vi "Begin.vi"(8 "error in":errorcluster) -> (0 "error out":errorcluster)   [LabVIEW 2016]
doc: "Called before other user functions, this VI is expected to open initial I/O refnums, load in file data, and do all program initialization. Notice that the <B>error out</B> terminal is simply used for data flow. Wiring it to other structures or subVIs ensures that this VI runs first."
uses:
  <vilib>/Rock Robotics/WPI/DriverStation/WPI_DriverStationRobotMode2.ctl
  <vilib>/Rock Robotics/WPI/SafetyOutput/WPI_SafetyOutputConfigMenu.ctl
  <vilib>/Rock Robotics/WPI/Joystick/WPI_JoystickDeviceEnum.ctl
  <vilib>/Rock Robotics/WPI/ThirdParty/CanMotor/TalonSRX/WPI_CANTalonSRX_APIControlMode.ctl
  <vilib>/Rock Robotics/WPI/Solenoid/WPI_SolenoidChannel.ctl
  <vilib>/Rock Robotics/SystemInterfaces/spilib/spi_bus.ctl
  <vilib>/Rock Robotics/WPI/ThirdParty/CanMotor/TalonSRX/WPI_CANTalonSRX_APIFeedbackSelect.ctl
  <vilib>/Rock Robotics/SystemInterfaces/DIO/FPGA_DIOChannel.ctl
  Robot Global Data.vi
  <vilib>/Rock Robotics/WPI/RobotDrive/WPI_RobotDriveOpen4MotorWithExistingMotors.vi
  <vilib>/Rock Robotics/WPI/Solenoid/WPI_SolenoidOpenDouble.vi
  <vilib>/Rock Robotics/WPI/Solenoid/WPI_SolenoidOpenSingle.vi
  <vilib>/Rock Robotics/WPI/Gyro/WPI_GyroXRS450_SPI_Open.vi
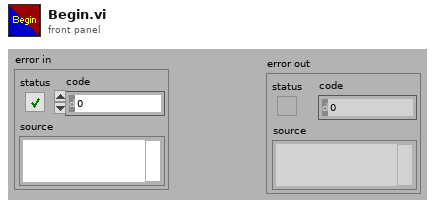
[diagram p1: front panel]
types:
  T1 = typedef "FPGA_DIOChannel.ctl" = enum8{"DIO 0", "DIO 1", "DIO 2", "DIO 3", "DIO 4", "DIO 5", "DIO 6", "DIO 7", "DIO 8", "DIO 9", "DIO MXP 0", "DIO MXP 1", "DIO MXP 2", "DIO MXP 3", "DIO MXP 4", "DIO MXP 5", "DIO MXP 6", "DIO MXP 7", "DIO MXP 8", "DIO MXP 9", "DIO MXP 10", "DIO MXP 11", "DIO MXP 12", "DIO MXP 13", "DIO MXP 14", "DIO MXP 15", "SPI Port CS1", "SPI Port CS2", "SPI Port CS3", "SPI Port MISO", "SPI Port MOSI", "Invalid"}
  T2 = typedef "WPI_CANTalonSRX_APIFeedbackSelect.ctl" = enum16{"Digital Quadrature Encoder", "Analog Potentiometer", "Analog Encoder", "Count on Quad-A (Rising-Edge)", "Count on Quad-A (Falling-Edge)", "CTR Magnetic Enc (Absolute)", "CTR Magnetic Enc (Relative)", "Pulse Width"}
  T3 = typedef "spi_bus.ctl" = enum16{"SPI On-Board, CS0", "SPI On-Board, CS1", "SPI On-Board, CS2", "SPI On-Board, CS3", "SPI MXP", "Invalid"}
  T4 = typedef "WPI_SolenoidChannel.ctl" = enum8{"Solenoid 0", "Solenoid 1", "Solenoid 2", "Solenoid 3", "Solenoid 4", "Solenoid 5", "Solenoid 6", "Solenoid 7", "Invalid"}
  T5 = typedef "WPI_CANTalonSRX_APIControlMode.ctl" = enum8{"Percent VBus", "Speed", "Position", "Slave", "Unchanged / Invalid", "Voltage Compensation", "Current", "Motion Profile", "Motion Magic"}
  T6 = typedef "WPI_JoystickDeviceEnum.ctl" = enum16{"USB 0", "USB 1", "USB 2", "USB 3", "USB 4", "USB 5"}
  T7 = typedef "WPI_SafetyOutputConfigMenu.ctl" = enum16{"Enable", "Disable"}
  T8 = typedef "WPI_DriverStationRobotMode2.ctl" = enum16{"Autonomous Disabled", "Autonomous Enabled", "Teleop Disabled", "Teleop Enabled", "Disconnected", "Finish", "Test Disabled", "Test Enabled", "Emergency Stopped"}
  T9 = typedef "WPI_JoystickDevRef.ctl" = cluster{"Device":T6}
  T10 = typedef "WPI_SolenoidDevRef.ctl" = cluster{"DevStatus":errorcluster, "Pneumatics Control Module":u8, "Forward Solenoid Channel":T4, "Reverse Solenoid Channel":T4}
  T11 = typedef "WPI_GyroDevRef.ctl" = cluster{"DevStatus":errorcluster, "Analog Channel":T12, "Offset":dbl, "Gain (VoltsPerDegree/Second)":dbl, "Gyro Type":enum16{"Analog", "XRS450"}, "Handle":i32, "SPI Bus":T3, "Device Found":bool, "Sample Rate":dbl, "Calibrate On Open":bool}
  T12 = typedef "FPGA_AIChannel.ctl" = enum8{"AI 0", "AI 1", "AI 2", "AI 3", "AI MXP 0", "AI MXP 1", "AI MXP 2", "AI MXP 3", "Invalid"}
  T13 = typedef "WPI_MotorControlDeviceRef.ctl" = cluster{"DeviceStatus":errorcluster, "Type":T14, "PWM":cluster{"PWM Channel":T15, "DeadBand":T16}, "CAN":cluster{"Device Number":u8, "SetOutput VI Ref":variant, "GetOutput VI Ref":variant, "Enable VI Ref":variant, "Disable VI Ref":variant, "Data":variant}, "Invert":bool}
  T14 = typedef "WPI_MotorControlType.ctl" = enum16{"PWM", "CAN"}
  T15 = typedef "FPGA_DIOPWMChannel.ctl" = enum8{"PWM 0", "PWM 1", "PWM 2", "PWM 3", "PWM 4", "PWM 5", "PWM 6", "PWM 7", "PWM 8", "PWM 9", "PWM MXP 0", "PWM MXP 1", "PWM MXP 2", "PWM MXP 3", "PWM MXP 4", "PWM MXP 5", "PWM MXP 6", "PWM MXP 7", "PWM MXP 8", "PWM MXP 9", "Invalid"}
  T16 = typedef "WPI_PWMDeadband.ctl" = cluster{"Name":string, "maxPositivePwm":i32, "minPositivePwm":i32, "centerPwm":i32, "maxNegativePwm":i32, "minNegativePwm":i32, "angularRange":u16}
  T17 = typedef "WPI_RobotDriveDevRef.ctl" = cluster{"DevStatus":errorcluster, "Motors[]":T13[], "Square Inputs":bool, "Max Output":dbl}
  T18 = typedef "WPI_DigitalOutputDevRef.ctl" = cluster{"DIO Channel":T1, "DevStatus":errorcluster}
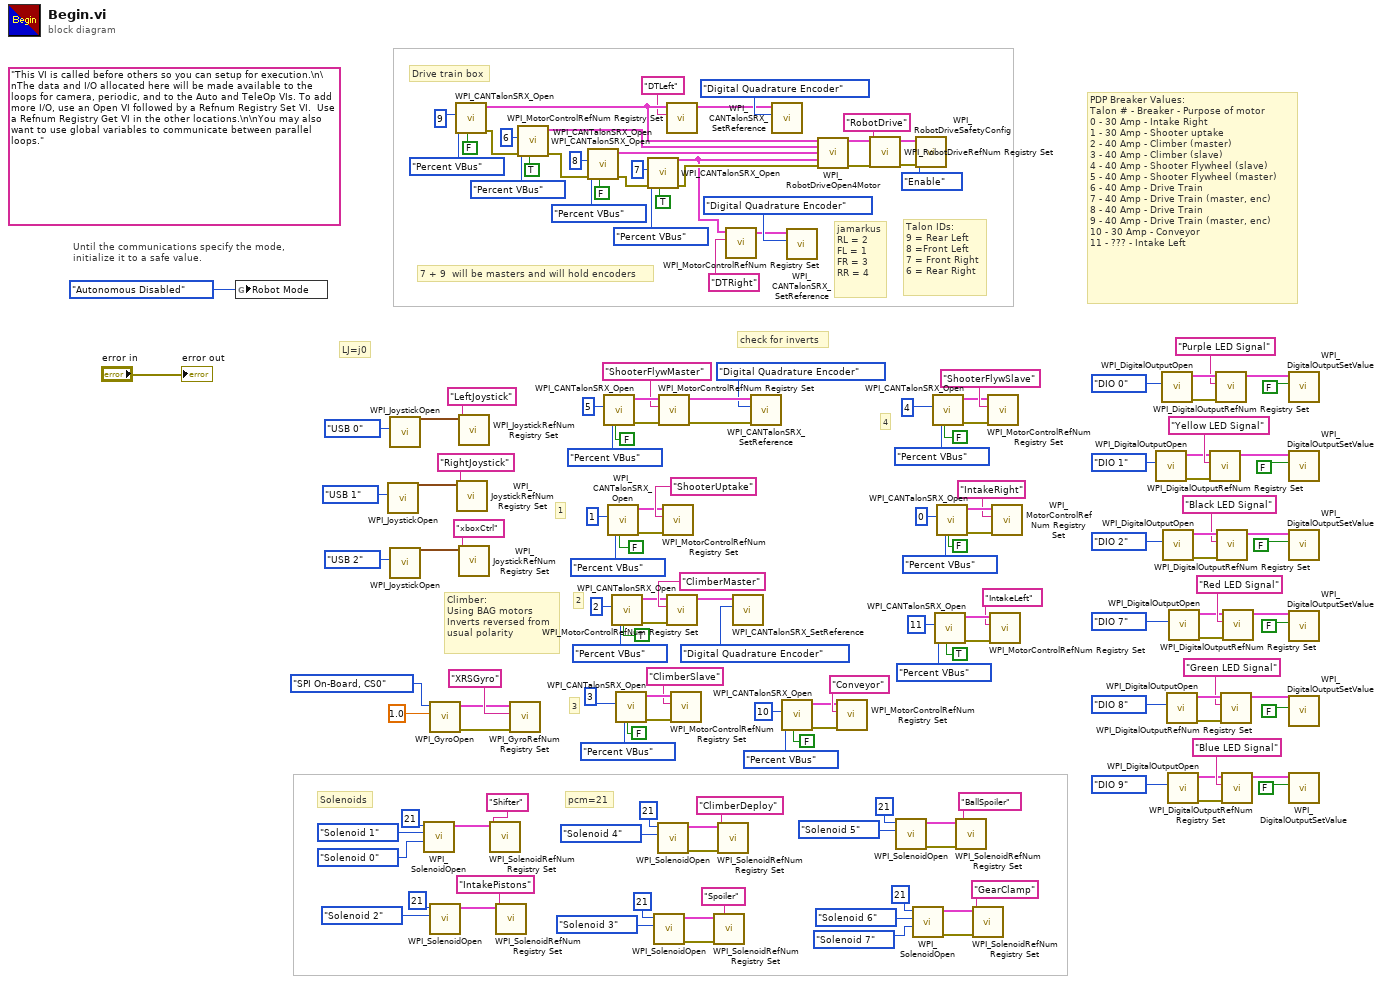
[diagram p0: block diagram]
diagram:
  (unwired) "This VI is called before others so you can setup for execution.\n\nThe data and I/O allocated here will be made available to the loops for camera, periodic, and to the Auto and TeleOp VIs. To add more I/O, use an Open VI followed by a Refnum Registry Set VI.  Use a Refnum Registry Get VI in the other locations.\n\nYou may also want to use global variables to communicate between parallel loops."
  # "3"
  # "2"
  # "1"
  # "4"
  # "jamarkus\nRL = 2\nFL = 1\nFR = 3\nRR = 4"
  # "pcm=21"
  # "Climber:\nUsing BAG motors\nInverts reversed from\nusual polarity"
  # "check for inverts"
  # "LJ=j0"
  # "PDP Breaker Values:\nTalon # - Breaker - Purpose of motor\n0 - 30 Amp - Intake Right\n1 - 30 Amp - Shooter uptake\n2 - 40 Amp - Climber (master)\n3 - 40 Amp - Climber (slave)\n4 - 40 Amp - Shooter Flywheel (slave)\n5 - 40 Amp - Shooter Flywheel (master)\n6 - 40 Amp - Drive Train\n7 - 40 Amp - Drive Train (master, enc)\n8 - 40 Amp - Drive Train\n9 - 40 Amp - Drive Train (master, enc)\n10 - 30 Amp - Conveyor\n11 - ??? - Intake Left"
  # "Solenoids"
  # "7 + 9  will be masters and will hold encoders"
  # "Talon IDs:\n9 = Rear Left\n8 =Front Left\n7 = Front Right\n6 = Rear Right"
  # "Drive train box"
  # "Until the communications specify the mode,\ninitialize it to a safe value."
  n1 = global write "Robot Global Data.vi" "Robot Mode"(WPI_DriverStationRobotMode2."Autonomous Disabled" ("Robot Mode")) -> ()
  n2 = call <vilib>:"WPI_JoystickOpen.vi"("JoystickDevice"=WPI_JoystickDeviceEnum."USB 1") -> ("JoystickDevRef"=w138:T9)  [unwired: 10 in]
  n3 = call <vilib>:"WPI_JoystickOpen.vi"("JoystickDevice"=WPI_JoystickDeviceEnum."USB 0") -> ("JoystickDevRef"=w141:T9)  [unwired: 10 in]
  n4 = call <vilib>:"WPI_JoystickOpen.vi"("JoystickDevice"=WPI_JoystickDeviceEnum."USB 2") -> ("JoystickDevRef"=w135:T9)  [unwired: 10 in]
  n5 = call-poly <vilib>:"WPI_SolenoidOpen.vi"("Reverse Solenoid Channel"=WPI_SolenoidChannel."Solenoid 0", "Forward Solenoid Channel"=WPI_SolenoidChannel."Solenoid 1", "Pneumatics Control Module (0)"=u8 21) -> ("SolenoidDevRef"=w98:T10)  [unwired: 7 in, 1 out]
  n6 = call-poly <vilib>:"WPI_GyroOpen.vi"("Sample Rate (ms)"=1.0, "SPI Bus"=spi_bus."SPI On-Board, CS0") -> ("error out"=w47:errorcluster, "GyroDevRef"=w46:T11)  [unwired: 8 in]
  n7 = call-poly <vilib>:"WPI_SolenoidOpen.vi"("Solenoid Channel"=WPI_SolenoidChannel."Solenoid 2" ("Reverse Solenoid Channel"), "Pneumatics Control Module (0)"=u8 21) -> ("SolenoidDevRef"=w91:T10)  [unwired: 8 in, 1 out]
  n8 = call <vilib>:"WPI_CANTalonSRX_Open.vi"("Invert"=FALSE, "Device Number"=u8 9, "Control Mode"=WPI_CANTalonSRX_APIControlMode."Percent VBus") -> ("error out"=w157:errorcluster, "CAN Talon SRX Ref"=w43:T13)  [unwired: 7 in]
  n9 = call <vilib>:"WPI_JoystickRefNum Registry Set.vi"("refnum name"="RightJoystick", "JoystickDevRef"=w138) -> ()  [unwired: 8 in, 2 out]
  n10 = call <vilib>:"WPI_JoystickRefNum Registry Set.vi"("refnum name"="LeftJoystick", "JoystickDevRef"=w141) -> ()  [unwired: 8 in, 2 out]
  n11 = call <vilib>:"WPI_JoystickRefNum Registry Set.vi"("refnum name"="xboxCtrl", "JoystickDevRef"=w135) -> ()  [unwired: 8 in, 2 out]
  n12 = call <vilib>:"WPI_SolenoidRefNum Registry Set.vi"("refnum name"="Shifter", "SolenoidDevRef"=w98) -> ()  [unwired: 8 in, 2 out]
  n13 = call <vilib>:"WPI_SolenoidRefNum Registry Set.vi"("refnum name"="IntakePistons", "SolenoidDevRef"=w91) -> ()  [unwired: 8 in, 2 out]
  n14 = call <vilib>:"WPI_GyroRefNum Registry Set.vi"("error in (no error)"=w47, "refnum name"="XRSGyro", "GyroDevRef"=w46) -> ()  [unwired: 7 in, 2 out]
  n15 = call <vilib>:"WPI_CANTalonSRX_Open.vi"("Invert"=TRUE, "error in"=w157, "Device Number"=u8 6, "Control Mode"=WPI_CANTalonSRX_APIControlMode."Percent VBus") -> ("error out"=w158:errorcluster, "CAN Talon SRX Ref"=w156:T13)  [unwired: 6 in]
  n16 = call <vilib>:"WPI_CANTalonSRX_Open.vi"("Invert"=FALSE, "error in"=w158, "Device Number"=u8 8, "Control Mode"=WPI_CANTalonSRX_APIControlMode."Percent VBus") -> ("error out"=w159:errorcluster, "CAN Talon SRX Ref"=w155:T13)  [unwired: 6 in]
  n17 = call <vilib>:"WPI_CANTalonSRX_Open.vi"("Invert"=FALSE, "Device Number"=u8 5, "Control Mode"=WPI_CANTalonSRX_APIControlMode."Percent VBus") -> ("error out"=w130:errorcluster, "CAN Talon SRX Ref"=w133:T13)  [unwired: 7 in]
  n18 = call <vilib>:"WPI_CANTalonSRX_Open.vi"("Invert"=FALSE, "Device Number"=u8 1, "Control Mode"=WPI_CANTalonSRX_APIControlMode."Percent VBus") -> ("error out"=w127:errorcluster, "CAN Talon SRX Ref"=w124:T13)  [unwired: 7 in]
  n19 = call <vilib>:"WPI_CANTalonSRX_Open.vi"("Invert"=TRUE, "Device Number"=u8 2, "Control Mode"=WPI_CANTalonSRX_APIControlMode."Percent VBus") -> ("error out"=w117:errorcluster, "CAN Talon SRX Ref"=w114:T13)  [unwired: 7 in]
  n20 = call <vilib>:"WPI_CANTalonSRX_Open.vi"("Invert"=FALSE, "Device Number"=u8 3, "Control Mode"=WPI_CANTalonSRX_APIControlMode."Percent VBus") -> ("error out"=w120:errorcluster, "CAN Talon SRX Ref"=w123:T13)  [unwired: 7 in]
  n21 = call <vilib>:"WPI_CANTalonSRX_Open.vi"("Invert"=TRUE, "error in"=w159, "Device Number"=u8 7, "Control Mode"=WPI_CANTalonSRX_APIControlMode."Percent VBus") -> ("error out"=w160:errorcluster, "CAN Talon SRX Ref"=w39:T13)  [unwired: 6 in]
  n22 = call-poly <vilib>:"WPI_SolenoidOpen.vi"("Solenoid Channel"=WPI_SolenoidChannel."Solenoid 3", "Pneumatics Control Module (0)"=u8 21) -> ("error out"=w53:errorcluster, "SolenoidDevRef"=w54:T10)  [unwired: 8 in]
  n23 = call-poly <vilib>:"WPI_SolenoidOpen.vi"("Solenoid Channel"=WPI_SolenoidChannel."Solenoid 4", "Pneumatics Control Module (0)"=u8 21) -> ("error out"=w80:errorcluster, "SolenoidDevRef"=w79:T10)  [unwired: 8 in]
  n24 = call <vilib>:"WPI_MotorControlRefNum Registry Set.vi"("error in (no error)"=w130, "refnum name"="ShooterFlywMaster", "MotorControlDevRef"=w133) -> ("error out"=w74:errorcluster, "MotorControlDevRef"=w73:T13)  [unwired: 7 in]
  n25 = call <vilib>:"WPI_MotorControlRefNum Registry Set.vi"("error in (no error)"=w127, "refnum name"="ShooterUptake", "MotorControlDevRef"=w124) -> ()  [unwired: 7 in, 2 out]
  n26 = call <vilib>:"WPI_MotorControlRefNum Registry Set.vi"("refnum name"="DTLeft", "MotorControlDevRef"=w43) -> ("MotorControlDevRef"=w41:T13)  [unwired: 8 in, 1 out]
  n27 = call <vilib>:"WPI_MotorControlRefNum Registry Set.vi"("error in (no error)"=w117, "refnum name"="ClimberMaster", "MotorControlDevRef"=w114) -> ("MotorControlDevRef"=w64:T13)  [unwired: 7 in, 1 out]
  n28 = call <vilib>:"WPI_MotorControlRefNum Registry Set.vi"("error in (no error)"=w120, "refnum name"="ClimberSlave", "MotorControlDevRef"=w123) -> ()  [unwired: 7 in, 2 out]
  n29 = call <vilib>:"WPI_SolenoidRefNum Registry Set.vi"("error in (no error)"=w53, "refnum name"="Spoiler", "SolenoidDevRef"=w54) -> ()  [unwired: 7 in, 2 out]
  n30 = call <vilib>:"WPI_SolenoidRefNum Registry Set.vi"("error in (no error)"=w80, "refnum name"="ClimberDeploy", "SolenoidDevRef"=w79) -> ()  [unwired: 7 in, 2 out]
  n31 = call <vilib>:"WPI_MotorControlRefNum Registry Set.vi"("refnum name"="DTRight", "MotorControlDevRef"=w39) -> ("MotorControlDevRef"=w40:T13)  [unwired: 8 in, 1 out]
  n32 = call <vilib>:"WPI_CANTalonSRX_SetReference.vi"("Feedback Reference"=WPI_CANTalonSRX_APIFeedbackSelect."Digital Quadrature Encoder", "CAN Talon SRX Ref"=w64) -> ()  [unwired: 8 in, 2 out]
  n33 = call <vilib>:"WPI_CANTalonSRX_SetReference.vi"("error in (no error)"=w74, "Feedback Reference"=WPI_CANTalonSRX_APIFeedbackSelect."Digital Quadrature Encoder", "CAN Talon SRX Ref"=w73) -> ()  [unwired: 7 in, 2 out]
  n34 = call <vilib>:"WPI_CANTalonSRX_SetReference.vi"("Feedback Reference"=WPI_CANTalonSRX_APIFeedbackSelect."Digital Quadrature Encoder", "CAN Talon SRX Ref"=w41) -> ()  [unwired: 8 in, 2 out]
  n35 = call <vilib>:"WPI_CANTalonSRX_Open.vi"("Invert"=FALSE, "Device Number"=u8 10, "Control Mode"=WPI_CANTalonSRX_APIControlMode."Percent VBus") -> ("error out"=w102:errorcluster, "CAN Talon SRX Ref"=w99:T13)  [unwired: 7 in]
  n36 = call <vilib>:"WPI_CANTalonSRX_SetReference.vi"("Feedback Reference"=WPI_CANTalonSRX_APIFeedbackSelect."Digital Quadrature Encoder", "CAN Talon SRX Ref"=w40) -> ()  [unwired: 8 in, 2 out]
  n37 = call-poly <vilib>:"WPI_RobotDriveOpen4Motor.vi"("Rear Left Motor Dev Ref"=w43, "Rear Right Motor Dev Ref"=w156, "Front Left Motor Dev Ref"=w155, "Front Right Motor Dev Ref"=w39, "error in (no error)"=w160) -> ("RobotDriveDevRef"=w166:T17, "error out"=w165:errorcluster)  [unwired: 9 in]
  n38 = call <vilib>:"WPI_MotorControlRefNum Registry Set.vi"("error in (no error)"=w102, "refnum name"="Conveyor", "MotorControlDevRef"=w99) -> ()  [unwired: 7 in, 2 out]
  n39 = call <vilib>:"WPI_RobotDriveRefNum Registry Set.vi"("error in (no error)"=w165, "refnum name"="RobotDrive", "RobotDriveDevRef"=w166) -> ("error out"=w164:errorcluster, "RobotDriveDevRef"=w163:T17)  [unwired: 7 in]
  n40 = call-poly <vilib>:"WPI_SolenoidOpen.vi"("Solenoid Channel"=WPI_SolenoidChannel."Solenoid 5", "Pneumatics Control Module (0)"=u8 21) -> ("error out"=w90:errorcluster, "SolenoidDevRef"=w89:T10)  [unwired: 8 in]
  n41 = call-poly <vilib>:"WPI_SolenoidOpen.vi"("Reverse Solenoid Channel"=WPI_SolenoidChannel."Solenoid 7", "Forward Solenoid Channel"=WPI_SolenoidChannel."Solenoid 6" ("Solenoid Channel"), "Pneumatics Control Module (0)"=u8 21) -> ("error out"=w81:errorcluster, "SolenoidDevRef"=w82:T10)  [unwired: 7 in]
  n42 = call <vilib>:"WPI_RobotDriveSafetyConfig.vi"("error in (no error)"=w164, "mode"=WPI_SafetyOutputConfigMenu."Enable", "RobotDriveDevRef"=w163) -> ()  [unwired: 7 in, 2 out]
  n43 = call <vilib>:"WPI_CANTalonSRX_Open.vi"("Invert"=FALSE, "Device Number"=u8 4, "Control Mode"=WPI_CANTalonSRX_APIControlMode."Percent VBus") -> ("error out"=w107:errorcluster, "CAN Talon SRX Ref"=w104:T13)  [unwired: 7 in]
  n44 = call <vilib>:"WPI_CANTalonSRX_Open.vi"("Invert"=TRUE, "Device Number"=u8 11, "Control Mode"=WPI_CANTalonSRX_APIControlMode."Percent VBus") -> ("error out"=w58:errorcluster, "CAN Talon SRX Ref"=w61:T13)  [unwired: 7 in]
  n45 = call <vilib>:"WPI_CANTalonSRX_Open.vi"("Invert"=FALSE, "Device Number"=u8 0, "Control Mode"=WPI_CANTalonSRX_APIControlMode."Percent VBus") -> ("error out"=w110:errorcluster, "CAN Talon SRX Ref"=w113:T13)  [unwired: 7 in]
  n46 = call <vilib>:"WPI_SolenoidRefNum Registry Set.vi"("error in (no error)"=w90, "refnum name"="BallSpoiler", "SolenoidDevRef"=w89) -> ()  [unwired: 7 in, 2 out]
  n47 = call <vilib>:"WPI_SolenoidRefNum Registry Set.vi"("error in (no error)"=w81, "refnum name"="GearClamp", "SolenoidDevRef"=w82) -> ()  [unwired: 7 in, 2 out]
  n48 = call <vilib>:"WPI_MotorControlRefNum Registry Set.vi"("error in (no error)"=w107, "refnum name"="ShooterFlywSlave", "MotorControlDevRef"=w104) -> ()  [unwired: 7 in, 2 out]
  n49 = call <vilib>:"WPI_MotorControlRefNum Registry Set.vi"("error in (no error)"=w58, "refnum name"="IntakeLeft", "MotorControlDevRef"=w61) -> ()  [unwired: 7 in, 2 out]
  n50 = call <vilib>:"WPI_MotorControlRefNum Registry Set.vi"("error in (no error)"=w110, "refnum name"="IntakeRight", "MotorControlDevRef"=w113) -> ()  [unwired: 7 in, 2 out]
  n51 = call <vilib>:"WPI_DigitalOutputOpen.vi"("DIO Channel"=FPGA_DIOChannel."DIO 1") -> ("error out"=w30:errorcluster, "DigitalOutputDevRef"=w31:T18)  [unwired: 9 in]
  n52 = call <vilib>:"WPI_DigitalOutputOpen.vi"("DIO Channel"=FPGA_DIOChannel."DIO 0") -> ("error out"=w37:errorcluster, "DigitalOutputDevRef"=w36:T18)  [unwired: 9 in]
  n53 = call <vilib>:"WPI_DigitalOutputOpen.vi"("DIO Channel"=FPGA_DIOChannel."DIO 2") -> ("error out"=w29:errorcluster, "DigitalOutputDevRef"=w28:T18)  [unwired: 9 in]
  n54 = call <vilib>:"WPI_DigitalOutputOpen.vi"("DIO Channel"=FPGA_DIOChannel."DIO 8") -> ("error out"=w21:errorcluster, "DigitalOutputDevRef"=w20:T18)  [unwired: 9 in]
  n55 = call <vilib>:"WPI_DigitalOutputOpen.vi"("DIO Channel"=FPGA_DIOChannel."DIO 9") -> ("error out"=w14:errorcluster, "DigitalOutputDevRef"=w15:T18)  [unwired: 9 in]
  n56 = call <vilib>:"WPI_DigitalOutputOpen.vi"("DIO Channel"=FPGA_DIOChannel."DIO 7") -> ("error out"=w22:errorcluster, "DigitalOutputDevRef"=w23:T18)  [unwired: 9 in]
  n57 = call <vilib>:"WPI_DigitalOutputRefNum Registry Set.vi"("error in (no error)"=w30, "refnum name"="Yellow LED Signal", "DigitalOutputDevRef"=w31) -> ("DigitalOutputDevRef"=w2:T18)  [unwired: 7 in, 1 out]
  n58 = call <vilib>:"WPI_DigitalOutputRefNum Registry Set.vi"("error in (no error)"=w37, "refnum name"="Purple LED Signal", "DigitalOutputDevRef"=w36) -> ("DigitalOutputDevRef"=w13:T18)  [unwired: 7 in, 1 out]
  n59 = call <vilib>:"WPI_DigitalOutputRefNum Registry Set.vi"("error in (no error)"=w29, "refnum name"="Black LED Signal", "DigitalOutputDevRef"=w28) -> ("DigitalOutputDevRef"=w3:T18)  [unwired: 7 in, 1 out]
  n60 = call <vilib>:"WPI_DigitalOutputRefNum Registry Set.vi"("error in (no error)"=w21, "refnum name"="Green LED Signal", "DigitalOutputDevRef"=w20) -> ("DigitalOutputDevRef"=w5:T18)  [unwired: 7 in, 1 out]
  n61 = call <vilib>:"WPI_DigitalOutputRefNum Registry Set.vi"("error in (no error)"=w14, "refnum name"="Blue LED Signal", "DigitalOutputDevRef"=w15) -> ("DigitalOutputDevRef"=w6:T18)  [unwired: 7 in, 1 out]
  n62 = call <vilib>:"WPI_DigitalOutputRefNum Registry Set.vi"("error in (no error)"=w22, "refnum name"="Red LED Signal", "DigitalOutputDevRef"=w23) -> ("DigitalOutputDevRef"=w4:T18)  [unwired: 7 in, 1 out]
  n63 = call <vilib>:"WPI_DigitalOutputSetValue.vi"("Value"=FALSE, "DigitalOutputDevRef"=w13) -> ()  [unwired: 8 in, 2 out]
  n64 = call <vilib>:"WPI_DigitalOutputSetValue.vi"("Value"=FALSE, "DigitalOutputDevRef"=w2) -> ()  [unwired: 8 in, 2 out]
  n65 = call <vilib>:"WPI_DigitalOutputSetValue.vi"("Value"=FALSE, "DigitalOutputDevRef"=w3) -> ()  [unwired: 8 in, 2 out]
  n66 = call <vilib>:"WPI_DigitalOutputSetValue.vi"("Value"=FALSE, "DigitalOutputDevRef"=w4) -> ()  [unwired: 8 in, 2 out]
  n67 = call <vilib>:"WPI_DigitalOutputSetValue.vi"("Value"=FALSE, "DigitalOutputDevRef"=w5) -> ()  [unwired: 8 in, 2 out]
  n68 = call <vilib>:"WPI_DigitalOutputSetValue.vi"("Value"=FALSE, "DigitalOutputDevRef"=w6) -> ()  [unwired: 8 in, 2 out]
  "error out" <- "error in"
